vi "Get Display String.vi"(11 "Test in":refnum<class "Test.lvclass">) -> (2 "Display String":string)   [LabVIEW 2018, in "Test.lvclass"]
uses:
  Test.lvclass
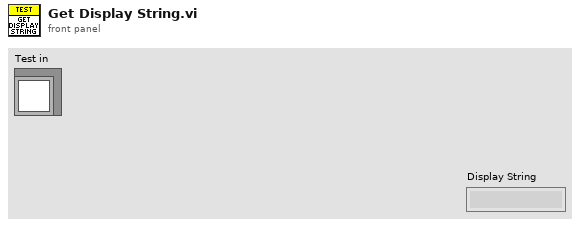
[diagram p1: front panel]
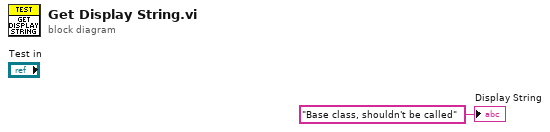
[diagram p0: block diagram]
diagram:
  "Display String" <- "Base class, shouldn't be called" ("Display String")
